vi "Send Command.vi"(8 "error in":errorcluster, 11 "MPLab in":refnum<class "MPLab.lvclass">) -> (0 "error out":errorcluster, 3 "MPLab out":refnum<class "MPLab.lvclass">)   [LabVIEW 2018, in "MPLab.lvlib" / "MPLab.lvclass"]
uses:
  MPLab.lvclass
  MPLab.lvclass/MPLab.ctl
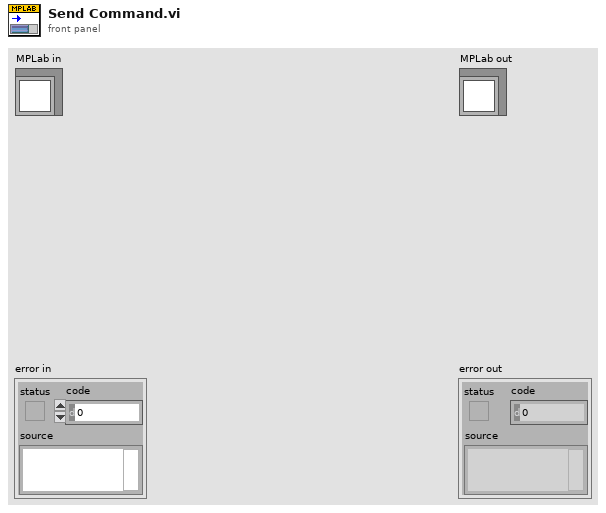
[diagram p1: front panel]
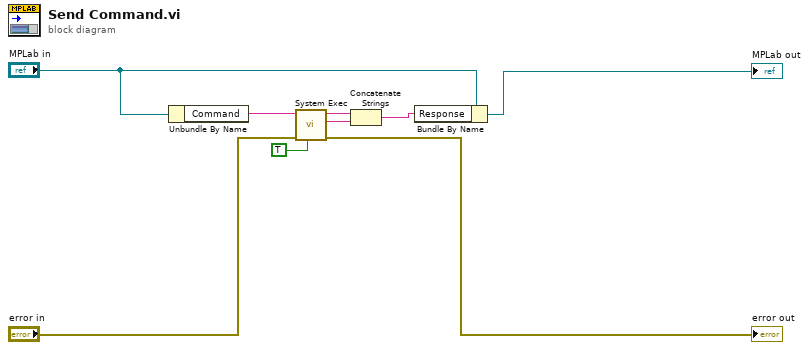
[diagram p0: block diagram]
diagram:
  n1 = Unbundle By Name("MPLab in") -> ("Command"=w9:string)
  n2 = call <vilib>:"System Exec.vi"("run minimized? (F)"=TRUE, "error in (no error)"="error in", "command line"=w9) -> ("error out"=→"error out":errorcluster, "standard error"=w2:string, "standard output"=w6:string)  [unwired: 5 in, 1 out]
  n3 = Concatenate Strings(w6, w2) -> (w3:string)
  n4 = Bundle By Name(cluster="MPLab in", "Response"=w3) -> (→"MPLab out":refnum<class "MPLab.lvclass">)
